vi "Heidenhain_Read.vi"(0 "VISA resource name out":refnum<visa-resource-name>, 1 "error out":errorcluster) -> (2 "VISA resource name out 2":refnum<visa-resource-name>, 3 "default value 1":dbl, 4 "error IO":errorcluster)   [LabVIEW 2009]
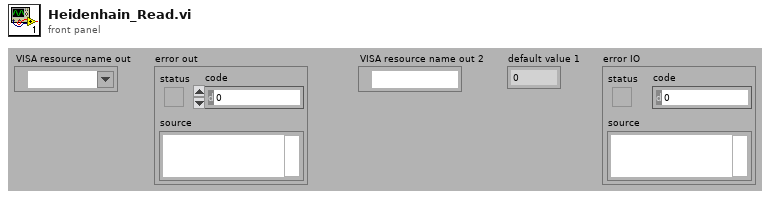
[diagram p1: front panel]
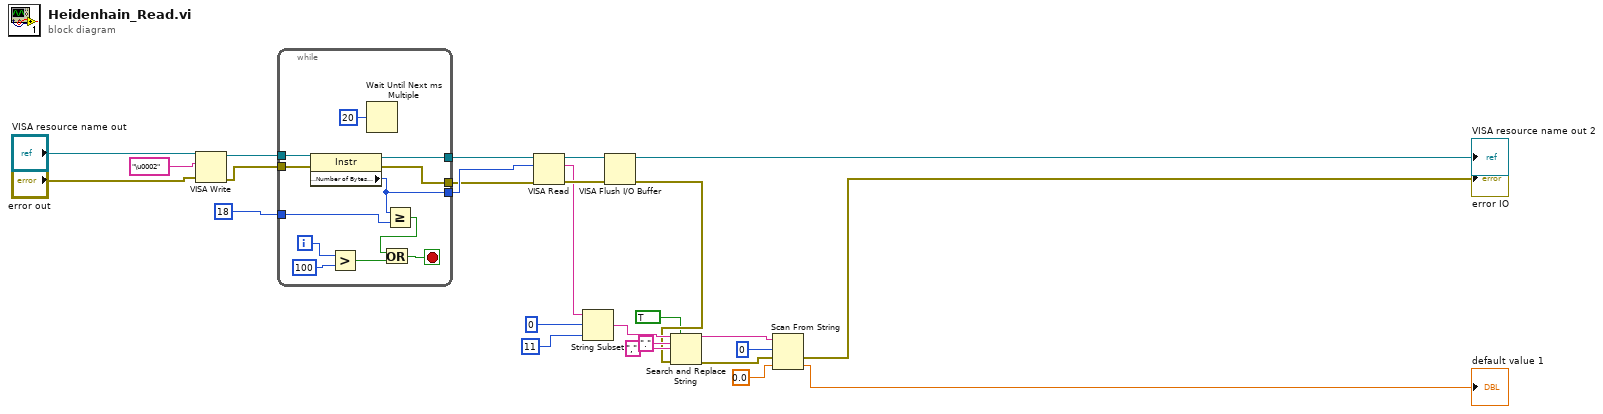
[diagram p0: block diagram]
diagram:
  n1 = VISA Write(VISA resource name="VISA resource name out", write buffer="\u0002", error in (no error)="error out") -> (VISA resource name out=w2:refnum<visa-resource-name>, error out=w3:errorcluster)  [unwired: 1 out]
  n2 = while {
    tunnel: w2 -> [w38]
    tunnel: w3 -> [w37]
    tunnel: [w36] -> w4
    tunnel: [w35] -> w5
    tunnel: [w34] -> w6
    tunnel: u32 18 ("y") -> [w28]
    i -> [w29]
    stop <- w32 stop-if-true
    n3 = property class="Instr"(reference=w38, error in=w37) -> (reference out=w36:refnum<visa-resource-name>, error out=w35:errorcluster, "Serial Settings:Number of Bytes at Serial Port"=w34:u32)
    n4 = Greater?(x=w29, y=100) -> (0:w30:bool)
    n5 = Wait Until Next ms Multiple(millisecond multiple=u32 20) -> ()  [unwired: 1 out]
    n6 = Greater Or Equal?(x=w34, y=w28) -> (x >= y?=w31:bool)
    n7 = Or(x=w31, y=w30) -> (x .or. y?=w32:bool)
  }
  n8 = VISA Read(VISA resource name=w4, byte count=w6, error in (no error)=w5) -> (VISA resource name out=w25:refnum<visa-resource-name>, read buffer=w21:string, error out=w24:errorcluster)  [unwired: 1 out]
  n9 = String Subset(string=w21, offset (0)=0, length (rest)=11 ("length (rest)")) -> (substring=w18:string)
  n10 = VISA Flush I/O Buffer(VISA resource name=w25, error in (no error)=w24) -> (VISA resource name out=→"VISA resource name out 2":refnum<visa-resource-name>, error out=w15:errorcluster)  [unwired: 1 out]
  n11 = Search and Replace String(replace all?=TRUE ("replace all? (F)"), input string=w18, search string=".", replace string="," ("replace string (\"\")"), error in=w15) -> (result string=w13:string, error out=w12:errorcluster)  [unwired: 5 out]
  n12 = Scan From String(input string=w13, initial scan location=u32 0, error in=w12, default 1=0.0 ("default value 1")) -> (error out=→"error IO":errorcluster, output 1=→"default value 1":dbl)  [unwired: 1 in, 2 out]
